vi "MoveState_Ex.vi"(4 "error in (no error)":errorcluster, 6 "Delay [ms]":i32=30 min=0, 7 "Control unit ID":i32=1 min=1 max=10) -> (0 "error out":errorcluster, 1 "Move state 3":i32, 2 "Move state 2":i32, 3 "Move state 1":i32)   [LabVIEW 2020]
panel:
  out "Axes state (123)":string
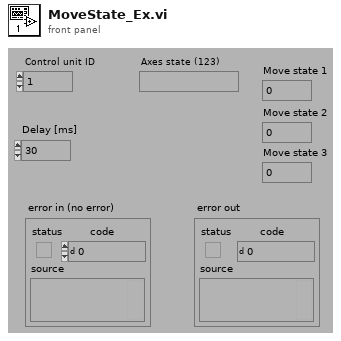
[diagram p1: front panel]
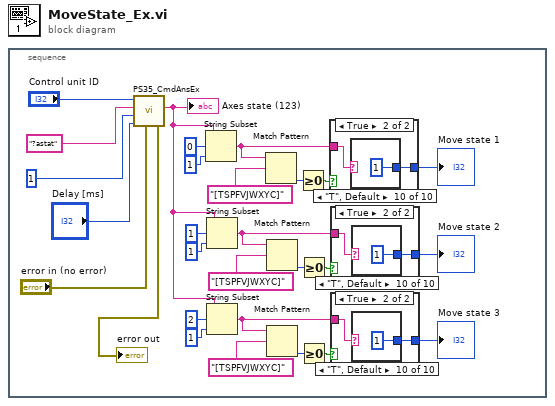
[diagram p0: block diagram]
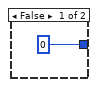
[diagram p2: hidden frame]
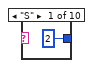
[diagram p3: hidden frame]
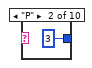
[diagram p4: hidden frame]
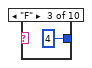
[diagram p5: hidden frame]
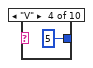
[diagram p6: hidden frame]
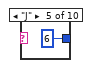
[diagram p7: hidden frame]
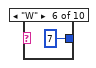
[diagram p8: hidden frame]
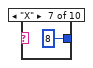
[diagram p9: hidden frame]
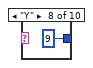
[diagram p10: hidden frame]
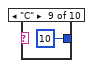
[diagram p11: hidden frame]
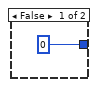
[diagram p12: hidden frame]
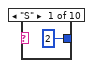
[diagram p13: hidden frame]
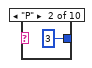
[diagram p14: hidden frame]
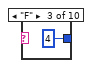
[diagram p15: hidden frame]
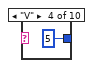
[diagram p16: hidden frame]
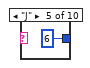
[diagram p17: hidden frame]
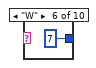
[diagram p18: hidden frame]
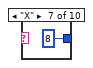
[diagram p19: hidden frame]
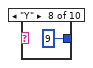
[diagram p20: hidden frame]
diagram:
  n1 = stacked-sequence {
    frame #0 {
      n2 = call "PS35_CmdAnsEx.vi"("error in (no error)"="error in (no error)", "nBreak"="Delay [ms]", "nRequest"=1, "Command"="?astat", "Control unit ID"="Control unit ID") -> ("error out"=→"error out":errorcluster, "Answer string"=w6:string)  [unwired: 2 in, 1 out]
      "Axes state (123)" <- w6
      n3 = String Subset(string=w6, offset (0)=0 ("Offset (0)"), length (rest)=1 ("Länge (Rest)")) -> (substring=w23:string)
      n4 = String Subset(string=w6, offset (0)=1 ("Offset (0)"), length (rest)=1 ("Länge (Rest)")) -> (substring=w15:string)
      n5 = String Subset(string=w6, offset (0)=2 ("Offset (0)"), length (rest)=1 ("Länge (Rest)")) -> (substring=w10:string)
      n6 = Match Pattern(string=w23, regular expression="[TSPFVJWXYC]" ("regulärer Ausdruck")) -> (offset past match=w21:i32)  [unwired: 1 in, 3 out]
      n7 = Match Pattern(string=w15, regular expression="[TSPFVJWXYC]" ("regulärer Ausdruck")) -> (offset past match=w17:i32)  [unwired: 1 in, 3 out]
      n8 = Match Pattern(string=w10, regular expression="[TSPFVJWXYC]" ("regulärer Ausdruck")) -> (offset past match=w8:i32)  [unwired: 1 in, 3 out]
      n9 = Greater Or Equal To 0?(x=w21) -> (x >= 0?=w20:bool)
      n10 = Greater Or Equal To 0?(x=w17) -> (x >= 0?=w18:bool)
      n11 = Greater Or Equal To 0?(x=w8) -> (x >= 0?=w7:bool)
      n12 = case shown="True" w20 {
        tunnel: w23 -> [_ w57]
        tunnel: [0 ("Länge (Rest)") w56] -> w19
        frame False {
        }
        frame True {
          n13 = case shown="\"T\", Default" w57 {
            tunnel: [2 ("Länge (Rest)") 3 ("Länge (Rest)") 4 ("Länge (Rest)") 5 ("Länge (Rest)") 6 ("Länge (Rest)") 7 ("Länge (Rest)") 8 ("Länge (Rest)") 9 ("Länge (Rest)") 10 ("Länge (Rest)") 1 ("Länge (Rest)")] -> w56
            frame "S" {
            }
            frame "P" {
            }
            frame "F" {
            }
            frame "V" {
            }
            frame "J" {
            }
            frame "W" {
            }
            frame "X" {
            }
            frame "Y" {
            }
            frame "C" {
            }
            frame "T", Default {
            }
          }
        }
      }
      "Move state 1" <- w19
      n14 = case shown="True" w18 {
        tunnel: w15 -> [_ w44]
        tunnel: [0 ("Länge (Rest)") w43] -> w5
        frame False {
        }
        frame True {
          n15 = case shown="\"T\", Default" w44 {
            tunnel: [2 ("Länge (Rest)") 3 ("Länge (Rest)") 4 ("Länge (Rest)") 5 ("Länge (Rest)") 6 ("Länge (Rest)") 7 ("Länge (Rest)") 8 ("Länge (Rest)") 9 ("Länge (Rest)") 10 ("Länge (Rest)") 1 ("Länge (Rest)")] -> w43
            frame "S" {
            }
            frame "P" {
            }
            frame "F" {
            }
            frame "V" {
            }
            frame "J" {
            }
            frame "W" {
            }
            frame "X" {
            }
            frame "Y" {
            }
            frame "C" {
            }
            frame "T", Default {
            }
          }
        }
      }
      "Move state 2" <- w5
      n16 = case shown="True" w7 {
        tunnel: w10 -> [_ w31]
        tunnel: [0 ("Länge (Rest)") w30] -> w4
        frame False {
        }
        frame True {
          n17 = case shown="\"T\", Default" w31 {
            tunnel: [2 ("Länge (Rest)") 3 ("Länge (Rest)") 4 ("Länge (Rest)") 5 ("Länge (Rest)") 6 ("Länge (Rest)") 7 ("Länge (Rest)") 8 ("Länge (Rest)") 9 ("Länge (Rest)") 10 ("Länge (Rest)") 1 ("Länge (Rest)")] -> w30
            frame "S" {
            }
            frame "P" {
            }
            frame "F" {
            }
            frame "V" {
            }
            frame "J" {
            }
            frame "W" {
            }
            frame "X" {
            }
            frame "Y" {
            }
            frame "C" {
            }
            frame "T", Default {
            }
          }
        }
      }
      "Move state 3" <- w4
    }
  }
